vi "Set Check Operation Data Status.vi"(7 "Register Value To Set (0)":i32, 8 "error in (no error)":errorcluster, 9 "Status Register Type (0: Enable Register)":i32(ring) items=["Enable Register", "Negative Transition Filter Register", "Positive Transition Filter Register", "Condition Register", "Event Register"], 10 "Operation Type (0: Check)":i32(ring) items=["Check", "Set"], 11 "VISA resource name":refnum<visa-resource-name>) -> (0 "error out":errorcluster, 2 "Register Status":bool[](array[boolean]), 3 "VISA resource name out":refnum<visa-resource-name>)   [LabVIEW 2017, in "Keysight B2980 Series.lvlib"]
doc: "Sets or checks the operation data status register.\n\n<B>Note(s):</B>\nUse this VI only with other low-level VIs. The high-level VIs automatically incorporate this functionality. This VI does not check the instrument status."
uses:
  Keysight B2980 Series.lvlib
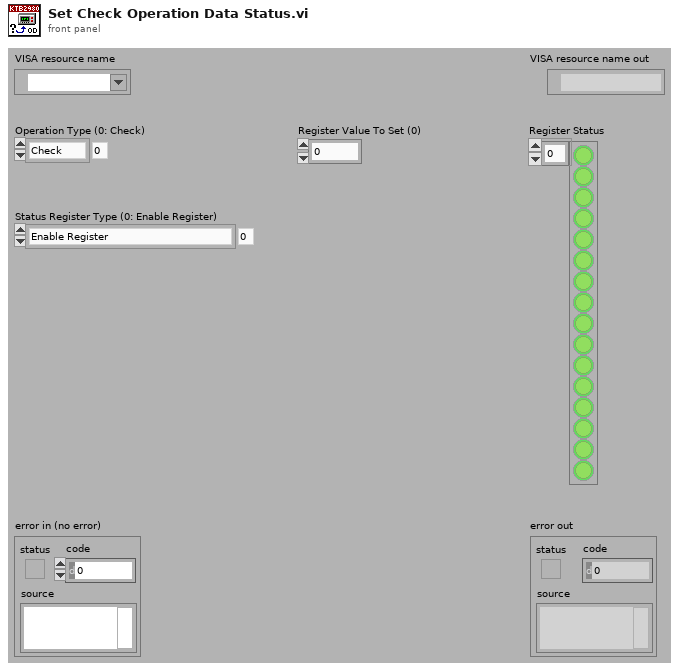
[diagram p1: front panel]
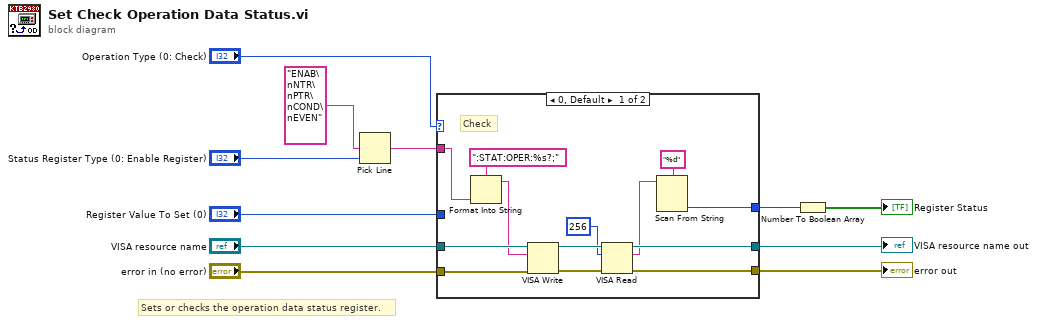
[diagram p0: block diagram]
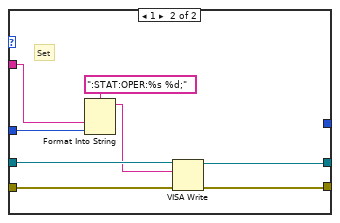
[diagram p2: hidden frame]
diagram:
  # "Sets or checks the operation data status register."
  n1 = Pick Line(multi-line string="ENAB\nNTR\nPTR\nCOND\nEVEN", line index="Status Register Type (0: Enable Register)") -> (output string=w10:string)  [unwired: 1 out]
  n2 = case shown="0, Default" "Operation Type (0: Check)" {
    tunnel: w10 -> [w23 w27]
    tunnel: "VISA resource name" -> [w22 w31]
    tunnel: "error in (no error)" -> [w21 w30]
    tunnel: [w16 w29] -> w9
    tunnel: [w15 w28] -> w8
    tunnel: [w12 _] -> w2
    tunnel: "Register Value To Set (0)" -> [_ w26]
    frame 0, Default {
      # "Check"
      n3 = Format Into String(format string=":STAT:OPER:%s?;", w23) -> (resulting string=w20:string)  [unwired: 2 in, 1 out]
      n4 = VISA Write(VISA resource name=w22, write buffer=w20, error in (no error)=w21) -> (VISA resource name out=w19:refnum<visa-resource-name>, error out=w18:errorcluster)  [unwired: 1 out]
      n5 = VISA Read(VISA resource name=w19, byte count=u32 256, error in (no error)=w18) -> (VISA resource name out=w16:refnum<visa-resource-name>, read buffer=w14:string, error out=w15:errorcluster)  [unwired: 1 out]
      n6 = Scan From String(format string="%d", input string=w14) -> (output 1=w12:i32)  [unwired: 2 in, 4 out]
    }
    frame 1 {
      # "Set"
      n7 = Format Into String(format string=":STAT:OPER:%s %d;", w27, w26) -> (resulting string=w25:string)  [unwired: 2 in, 1 out]
      n8 = VISA Write(VISA resource name=w31, write buffer=w25, error in (no error)=w30) -> (VISA resource name out=w29:refnum<visa-resource-name>, error out=w28:errorcluster)  [unwired: 1 out]
    }
  }
  "VISA resource name out" <- w9
  "error out" <- w8
  n9 = Number To Boolean Array(number=w2) -> (Boolean array=→"Register Status":bool[])
